vi "DataStream_PC_Add Point To Map.vi"(8 "Value":dbl, 9 "Time Stamp":dbl, 10 "Name":string, 11 "Map":map{string, T1}(c390)) -> (3 "Map Out":map{string, T1}(c390))   [LabVIEW 2020]
uses:
  TypeDefs/Cluster_DataStream PC Map Data Set.ctl
  <vilib>/Utility/miscctls.llb/LVMapReplaceAction.ctl
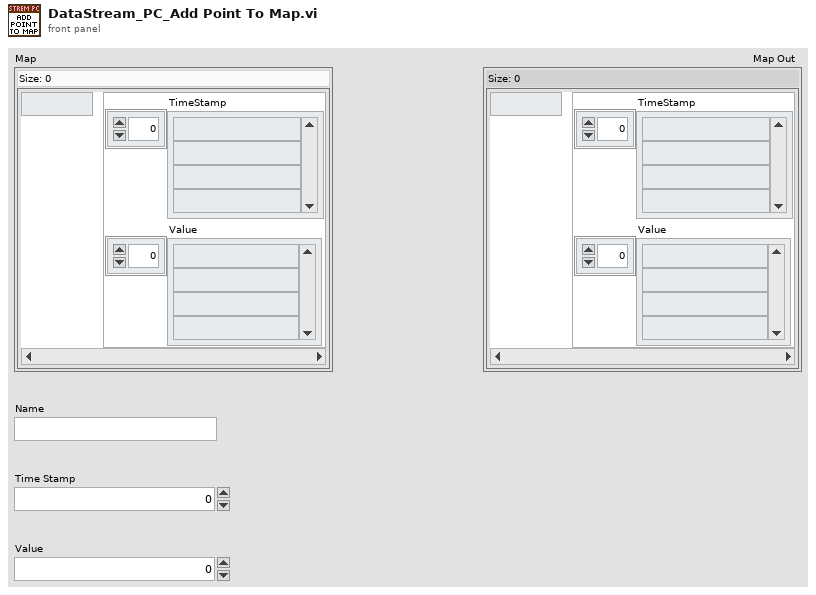
[diagram p1: front panel]
types:
  T1 = typedef "Cluster_DataStream PC Map Data Set.ctl" = cluster{"TimeStamp":dbl[], "Value":dbl[]}
  T2 = typedef "LVMapReplaceAction.ctl" = enum32{"Modify Entry only if found", "Add or Modify Entry", "Delete Entry"}
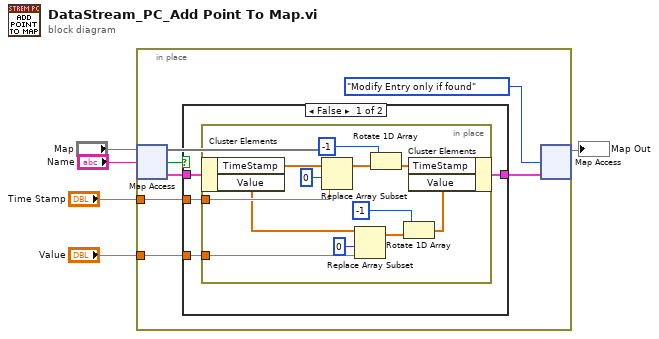
[diagram p0: block diagram]
diagram:
  n1 = in-place {
    in-place-border: "Time Stamp" -> [w10]
    in-place-border: "Value" -> [w9]
    n2 = in-place-map #1("Map", "Name") -> (w11:T1, w6:bool)  [unwired: 1 in]
    n3 = case shown="False" w6 {
      tunnel: w11 -> [w15 w28]
      tunnel: w10 -> [w14 _]
      tunnel: w9 -> [w13 _]
      tunnel: [w12 w28] -> w8
      frame False {
        n4 = in-place {
          in-place-border: w14 -> [w27]
          in-place-border: w13 -> [w26]
          n5 = in-place-cluster #2(w15) -> ("TimeStamp"=w23:dbl[], "Value"=w16:dbl[])
          n6 = Replace Array Subset(array=w23, new element=w27, index=0) -> (w22:dbl[])
          n7 = Replace Array Subset(array=w16, new element=w26, index=0) -> (w17:dbl[])
          n8 = Rotate 1D Array(1:w22, 2:-1 ("n")) -> (0:w24:dbl[])
          n9 = Rotate 1D Array(1:w17, 2:-1 ("n")) -> (0:w25:dbl[])
          n10 = in-place-cluster #2("TimeStamp"=w24, "Value"=w25) -> (w12:T1)
        }
      }
      frame True {
      }
    }
    n11 = in-place-map #1(w8, LVMapReplaceAction."Modify Entry only if found" ("action")) -> (→"Map Out":map{string, T1})  [unwired: 2 out]
  }
